vi "Configure Analog Gen Sine.vi"(0 "VISA resource name":refnum<visa-resource-name>, 1 "Frequency (10 Hz)":dbl=10.0, 2 "Enable Sine Waveform (T: Enable)":bool=TRUE, 5 "Channel (0: A)":i32(ring) items=["A", "B"], 7 "Sine Type (0: Sine)":i32(ring) items=["Sine", "LoDistSine", "PhasedSine"], 9 "Amplitude (0 Vrms)":dbl, 11 "error in (no error)":errorcluster, 12 "Enable EQ Output Modification (T: Enable)":bool=TRUE, 13 "Phase Difference (0 degrees)":dbl) -> (4 "VISA resource name out":refnum<visa-resource-name>, 15 "error out":errorcluster)   [LabVIEW 2014, in "Stanford Research SR1.lvlib"]
doc: "Configures the attributes for the Analog Generator Sine waveform."
uses:
  Stanford Research SR1.lvlib
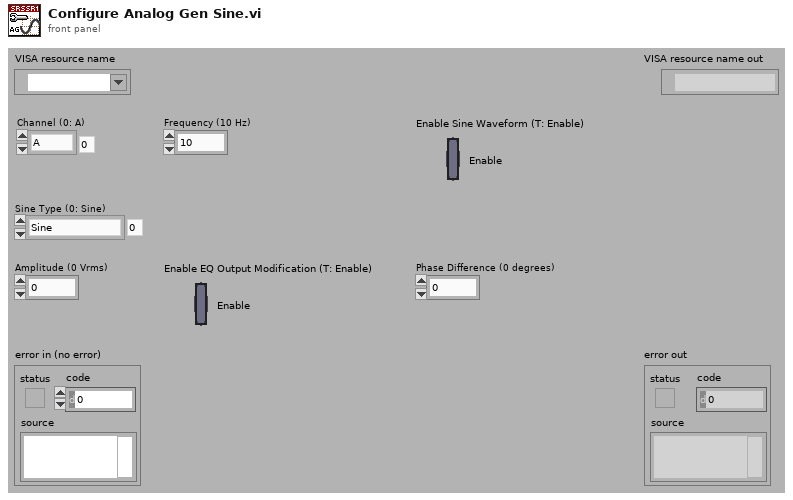
[diagram p1: front panel]
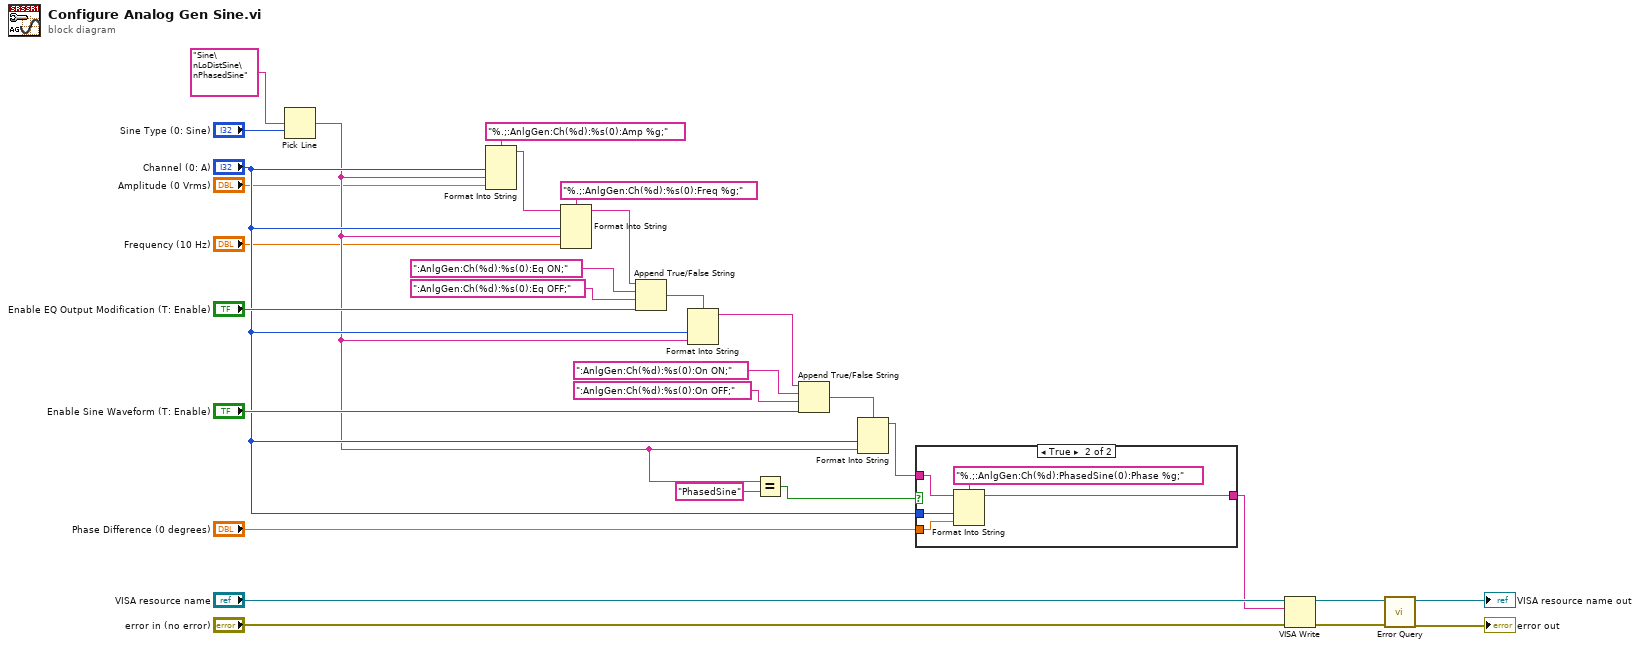
[diagram p0: block diagram]
diagram:
  n1 = Pick Line(multi-line string="Sine\nLoDistSine\nPhasedSine", line index="Sine Type (0: Sine)") -> (output string=w5:string)  [unwired: 1 in]
  n2 = Format Into String(format string="%.;:AnlgGen:Ch(%d):%s(0):Amp %g;", "Channel (0: A)", w5, "Amplitude (0 Vrms)") -> (resulting string=w11:string)  [unwired: 2 in, 1 out]
  n3 = Format Into String(format string="%.;:AnlgGen:Ch(%d):%s(0):Freq %g;", initial string=w11, "Channel (0: A)", w5, "Frequency (10 Hz)") -> (resulting string=w10:string)  [unwired: 1 in, 1 out]
  n4 = Append True/False String(1:"Enable EQ Output Modification (T: Enable)", 2:":AnlgGen:Ch(%d):%s(0):Eq OFF;", 3:":AnlgGen:Ch(%d):%s(0):Eq ON;", 4:w10) -> (0:w13:string)
  n5 = Format Into String(format string=w13, "Channel (0: A)", w5) -> (resulting string=w12:string)  [unwired: 2 in, 1 out]
  n6 = Equal?(x=w5, y="PhasedSine") -> (x = y?=w3:bool)
  n7 = Append True/False String(1:"Enable Sine Waveform (T: Enable)", 2:":AnlgGen:Ch(%d):%s(0):On OFF;", 3:":AnlgGen:Ch(%d):%s(0):On ON;", 4:w12) -> (0:w14:string)
  n8 = Format Into String(format string=w14, "Channel (0: A)", w5) -> (resulting string=w7:string)  [unwired: 2 in, 1 out]
  n9 = case shown="True" w3 {
    tunnel: "Channel (0: A)" -> [_ w35]
    tunnel: "Phase Difference (0 degrees)" -> [_ w32]
    tunnel: w7 -> [w31 w34]
    tunnel: [w31 w33] -> w6
    frame False {
    }
    frame True {
      n10 = Format Into String(format string="%.;:AnlgGen:Ch(%d):PhasedSine(0):Phase %g;", initial string=w34, w35, w32) -> (resulting string=w33:string)  [unwired: 1 in, 1 out]
    }
  }
  n11 = VISA Write(VISA resource name="VISA resource name", write buffer=w6, error in (no error)="error in (no error)") -> (VISA resource name out=w20:refnum<visa-resource-name>, error out=w19:errorcluster)  [unwired: 1 out]
  n12 = call "Error Query.vi"("error in (no error)"=w19, "VISA resource name"=w20) -> ("error out"=→"error out":errorcluster, "VISA resource name out"=→"VISA resource name out":refnum<visa-resource-name>)  [unwired: 6 in, 2 out]
